vi "NGTS_AO Parse Dbls to Tasks.vi"(8 "error in":errorcluster, 9 "AO Commands":dbl[](array[numeric]), 11 "AO Tasks In":refnum<k21>[](array[refnum])) -> (0 "error out":errorcluster, 2 "Array":cluster{"AO Commands":dbl[]}[](array[cluster]), 3 "AO Tasks Out":refnum<k21>[](array[refnum]))   [LabVIEW 2018]
uses:
  <resource>/objmgr/daqmx.rc
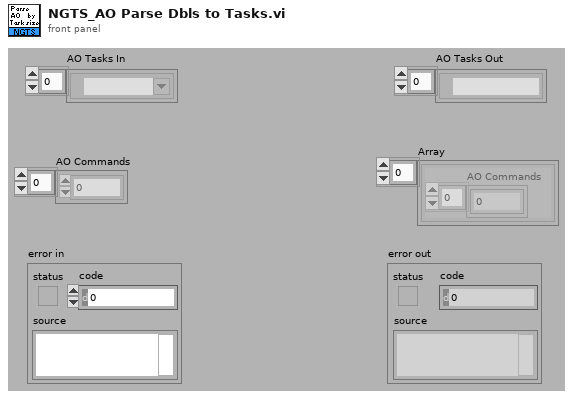
[diagram p1: front panel]
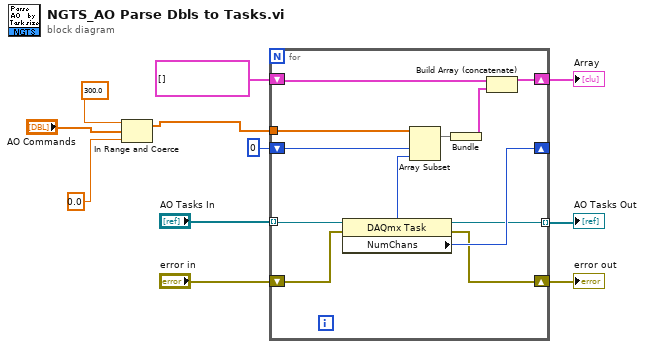
[diagram p0: block diagram]
diagram:
  n1 = In Range and Coerce(upper limit=300.0, x="AO Commands", lower limit=0.0) -> (coerced(x)=w1:dbl[])  [unwired: 1 out]
  n2 = for {
    tunnel: "AO Tasks In" -> [w22] mode=indexing
    shift-right: [w12] -> w9
    shift-left: "error in" -> [w13]
    shift-right: [w20] -> _
    shift-left: 0 -> [w21]
    tunnel: [w19] -> w7 mode=indexing
    tunnel: w1 -> [w18]
    shift-right: [w14] -> w6
    shift-left: cluster{"AO Commands":dbl[]}[] [] ("Array") -> [w16]
    n3 = property class="DAQmx Task"(reference=w22, error in=w13) -> (reference out=w19:refnum<k21>, error out=w12:errorcluster, "NumChans"=w20:u32)
    n4 = Array Subset(array=w18, index=w21, length=w20) -> (w17:dbl[])
    n5 = Bundle(w17) -> (w15:cluster{dbl[]})  [unwired: 1 in]
    n6 = Build Array (concatenate)(w16, w15) -> (w14:cluster{"AO Commands":dbl[]}[])
  }
  "Array" <- w6
  "AO Tasks Out" <- w7
  "error out" <- w9
